vi "Float_diag_state_space.vi"(5 "TF Order":i32=2, 7 "A_diag":sgl[](array[numeric])=[0.982758, -1.98194, 1.0, 0.0, 0.0, 0.0, 0.0, 0.0, 0.0], 8 "C":sgl[](array[numeric])=[-0.00254, 0.000408, 0.00295, 0.0, 0.0, 0.0, 0.0, 0.0, 0.0], 9 "State In":sgl[](array[numeric])=[0.0, 0.0, 0.0, 0.0, 0.0, 0.0, 0.0, 0.0, 0.0], 10 "Input":sgl) -> (2 "State Out":sgl[](array[numeric]), 3 "Output":sgl)   [LabVIEW 2017]
panel:
  in  "d":sgl
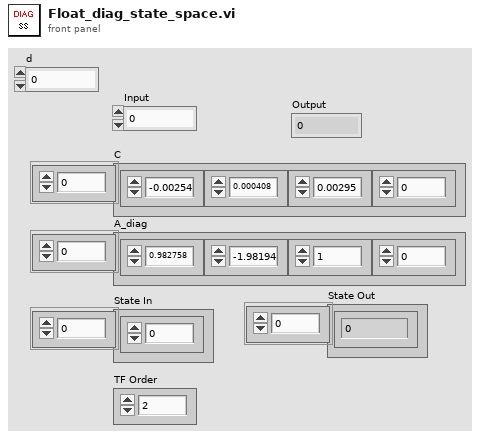
[diagram p1: front panel]
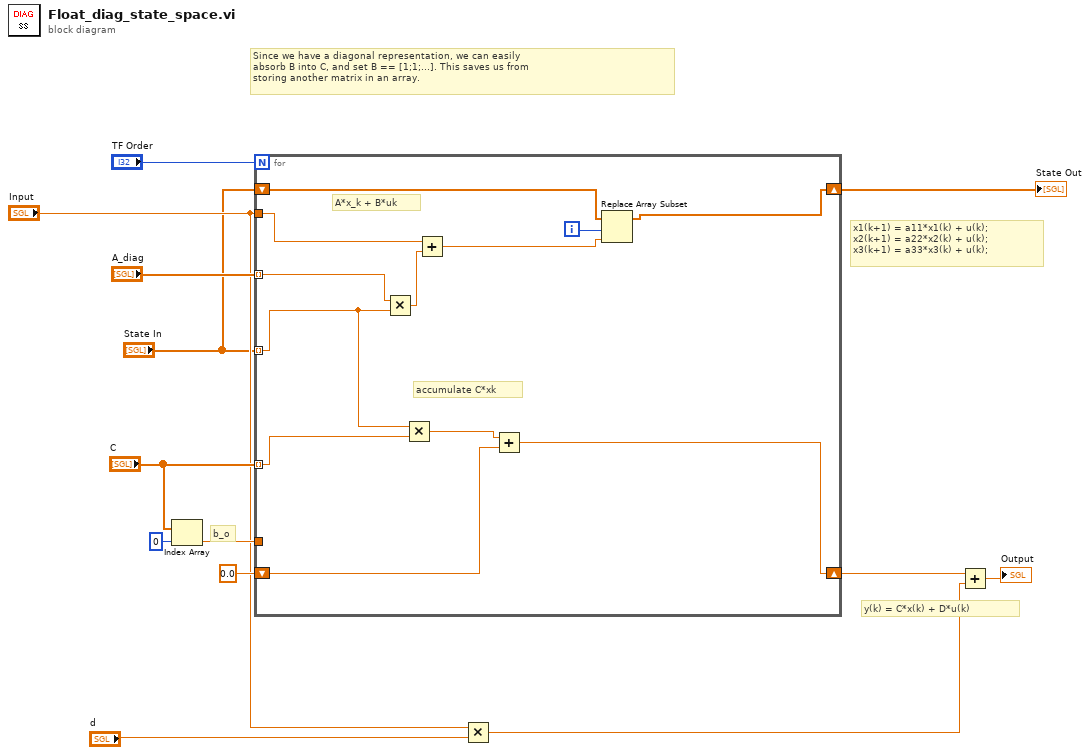
[diagram p0: block diagram]
diagram:
  # "Since we have a diagonal representation, we can easily\nabsorb B into C, and set B == [1;1;...]. This saves us from \nstoring another matrix in an array."
  # "x1(k+1) = a11*x1(k) + u(k);\nx2(k+1) = a22*x2(k) + u(k);\nx3(k+1) = a33*x3(k) + u(k);"
  # "y(k) = C*x(k) + D*u(k)"
  # "b_o"
  n1 = Index Array(array="C", index=0) -> (element=w10:sgl)
  n2 = for {
    N: "TF Order" -> [_]
    tunnel: "A_diag" -> [w25] mode=indexing
    tunnel: "C" -> [w23] mode=indexing
    shift-right: [w21] -> w5
    shift-left: sgl 0.0 ("element") -> [w20]
    tunnel: "Input" -> [w19]
    tunnel: w10 -> [_]
    tunnel: "State In" -> [w24] mode=indexing
    shift-right: [w14] -> w1
    shift-left: "State In" -> [w17]
    i -> [w16]
    # "accumulate C*xk"
    # "A*x_k + B*uk"
    n3 = Multiply(x=w25, y=w24) -> (x*y=w18:sgl)
    n4 = Multiply(x=w24, y=w23) -> (x*y=w22:sgl)
    n5 = Add(x=w19, y=w18) -> (x+y=w15:sgl)
    n6 = Add(x=w22, y=w20) -> (x+y=w21:sgl)
    n7 = Replace Array Subset(array=w17, new element=w15, index=w16) -> (w14:sgl[])
  }
  "State Out" <- w1
  n8 = Multiply(x="Input", y="d") -> (x*y=w3:sgl)
  n9 = Add(x=w5, y=w3) -> (x+y=→"Output":sgl)
